vi "SwitchBoard_ToggleDisplay.vi"(8 "error in":errorcluster, 10 "On/Off":bool, 11 "Handle":u32) -> (0 "error out":errorcluster, 3 "Handle out":u32)   [LabVIEW 2016]
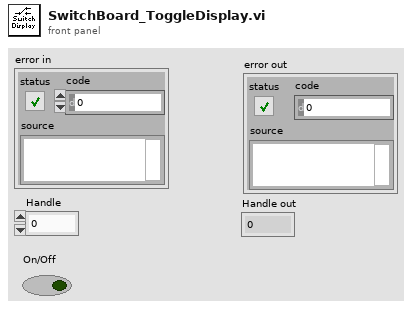
[diagram p1: front panel]
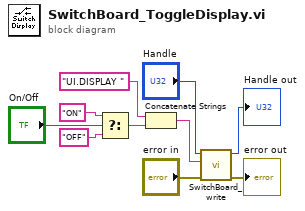
[diagram p0: block diagram]
diagram:
  n1 = Select(t="ON" ("string"), s="On/Off", f="OFF" ("string")) -> (s? t:f=w1:string)
  n2 = Concatenate Strings("UI.DISPLAY " ("string"), w1) -> (w9:string)
  n3 = call "SwitchBoard_write.vi"("error in"="error in", "Buffer"=w9, "Handle"="Handle") -> ("error out"=→"error out":errorcluster, "Handle"=→"Handle out":u32)  [unwired: 6 in, 1 out]
